vi "SPI IO port test.vi"() -> ()   [LabVIEW 2012]
uses:
  <vilib>/rvi/eio/common/nirviEmuTemplateMethod_errors.vi
  <vilib>/eio/EIONode/EIONode.xnode
panel:
  out "IO Read":bool
  in  "stop":bool
  in  "IO Write":bool
  in  "Action":enum16{"write", "read", ""}(ring)
  in  "FPGA I/O In":refnum<k21>="DIO17"
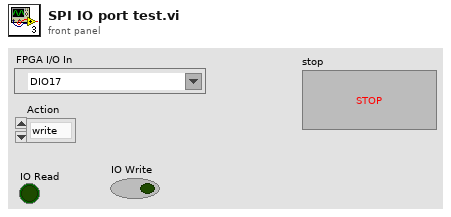
[diagram p1: front panel]
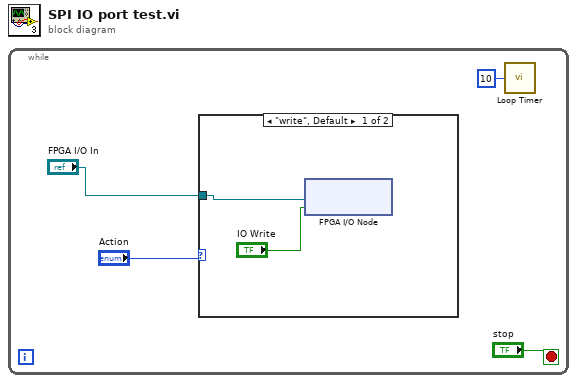
[diagram p0: block diagram]
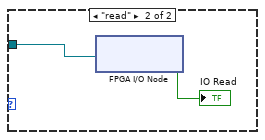
[diagram p2: hidden frame]
diagram:
  n1 = while {
    stop <- "stop" stop-if-true
    n2 = case shown="\"write\", Default" "Action" {
      tunnel: "FPGA I/O In" -> [w6 w8]
      frame "write", Default {
        n3 = xnode "FPGA I/O Node"("I/O Item"="IO Write", "FPGA I/O In"=w6) -> ()  [unwired: 1 out]
      }
      frame "read" {
        n4 = xnode "FPGA I/O Node"("FPGA I/O In"=w8) -> ("I/O Item"=→"IO Read":bool)  [unwired: 1 out]
      }
    }
    n5 = call "Loop Timer"("Count(mSec)"=u32 10) -> ()  [unwired: 1 out]
  }
